vi "Initialize.vi"(8 "error in":errorcluster, 11 "PCAP Frame Logger in":refnum<class "PCAP Frame Logger.lvclass">) -> (0 "error out":errorcluster, 3 "PCAP Frame Logger out":refnum<class "PCAP Frame Logger.lvclass">)   [LabVIEW 2020, in "Frame Logging.lvlib" / "PCAP Frame Logger.lvclass"]
uses:
  PCAP Frame Logger.lvclass
  PCAP Frame Logger.lvclass/PCAP Frame Logger.ctl
  libpcaplv/libpcaplv.lvlib
  <vilib>/nisyscfg/nisyscfg.lvlib
  <vilib>/Utility/SystemLogging/NI_SystemLogging.lvlib
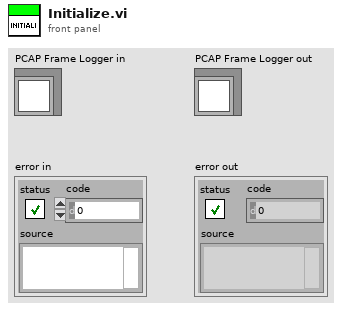
[diagram p1: front panel]
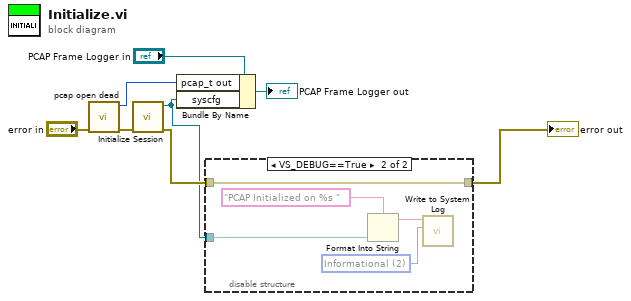
[diagram p0: block diagram]
diagram:
  n1 = call "pcap open dead.vi"("error in"="error in") -> ("error out"=w4:errorcluster, "pcap_t"=w5:u64)  [unwired: 9 in]
  n2 = call <vilib>:"Initialize Session.vi"("error in (no error)"=w4) -> ("error out"=w3:errorcluster, "Session out"=w1:refnum<k21>)  [unwired: 9 in]
  n3 = Bundle By Name(cluster="PCAP Frame Logger in", "pcap_t out"=w5, "syscfg"=w1) -> (→"PCAP Frame Logger out":refnum<class "PCAP Frame Logger.lvclass">)
  n4 = disable-structure shown="VS_DEBUG==True" {
    disable-tunnel: w3 -> [_ w10]
    disable-tunnel: [_ w10] -> w2
    disable-tunnel: w1 -> [_ w9]
    frame condition #0 (active) {
    }
    frame condition #1 {
      w11 = 2 items=["Error", "Warning", "Informational"] ("severity")
      n5 = Format Into String(format string="PCAP Initialized on %s ", w9) -> (resulting string=w12:string)  [unwired: 2 in, 1 out]
      n6 = call <vilib>:"Write to System Log.vi"("severity"=w11, "message"=w12) -> ()  [unwired: 9 in, 1 out]
    }
  }
  "error out" <- w2
